vi "Logging.vi"(8 "error in (no error)":errorcluster, 11 "Node Ptr":T1 format="%.0x") -> (0 "error out":errorcluster)   [LabVIEW 2020, in "Ballard ARINC 429 System Explorer.lvlib" / "Implementation.lvlib"]
uses:
  Implementation.lvlib
  <vilib>/NI VeriStand/Custom Device API/Custom Device API.lvlib
  Scripting/Ballard/Ballard ARINC 429 Scripting.lvlib
  <vilib>/NI VeriStand/Custom Device API/Custom Device Item Ref.ctl
panel:
  in  "Log Messages?":bool
  in  "Log Directory":string
  in  "SHDocVw.IWebBrowser":refnum<k7>(container)
  in  "General Header":cluster{"Section Name":string}={"Section Name"="Ballard ARINC 429 - Logging"}
  in  "Description":string
  out "Name":string
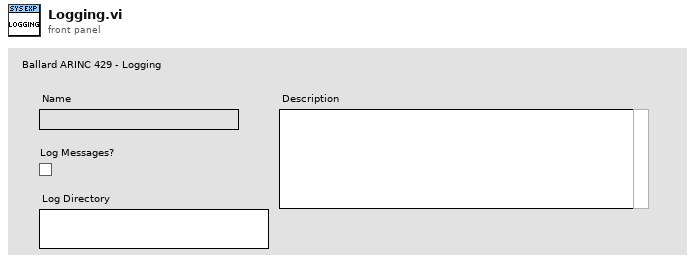
[diagram p1: front panel]
types:
  T1 = typedef "Custom Device API.lvlib/Custom Device Item Ref.ctl" = u64
  T2 = typedef "Custom Device API.lvlib/Custom Device Item Info.ctl" = cluster{"Name":string, "Is Channel":bool, "GUID":string, "Is Waveform":bool}
  T3 = typedef "Custom Device API.lvlib/Custom Device Commands.ctl" = enum16{"Default", "Item renamed", "Shutdown", "Dynamic button pressed"}
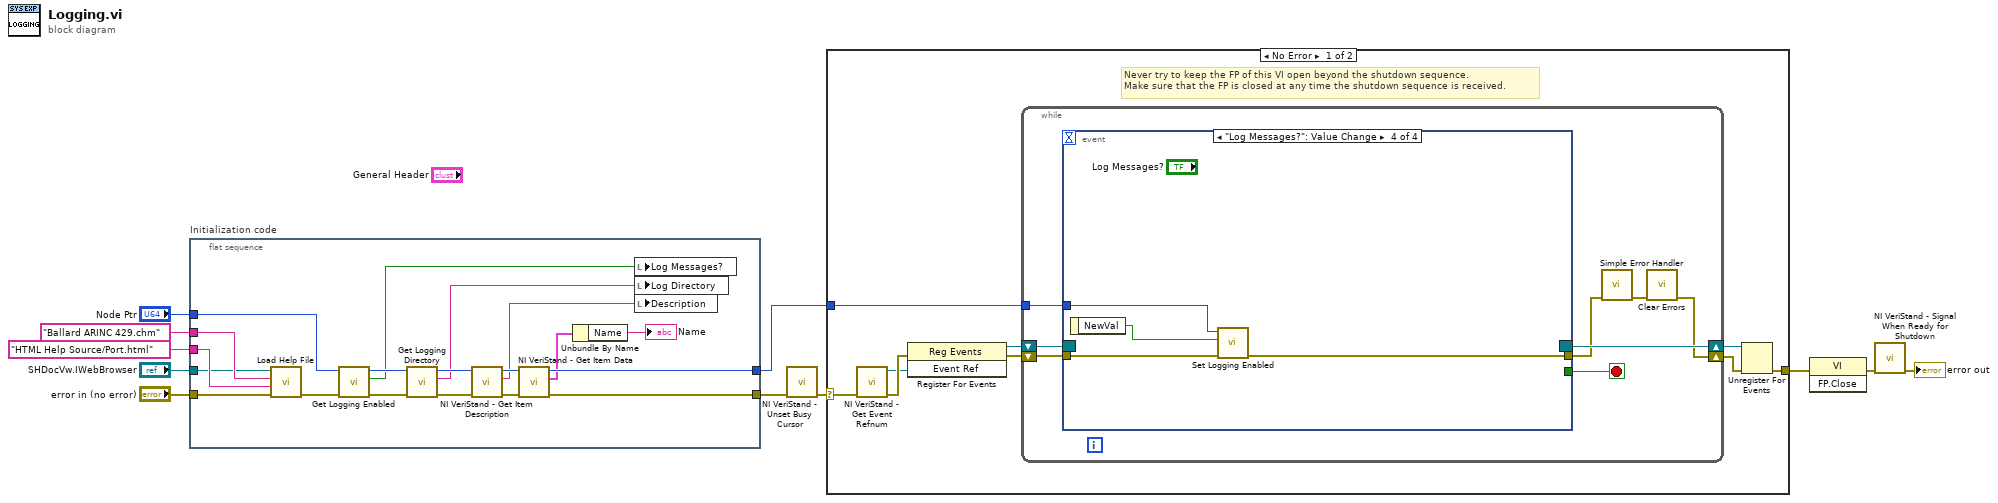
[diagram p0: block diagram]
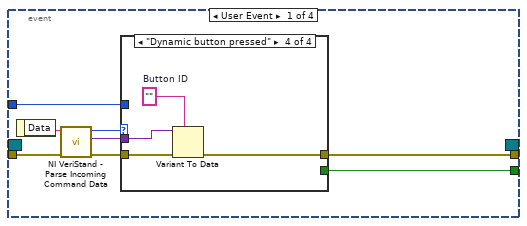
[diagram p2: hidden frame]
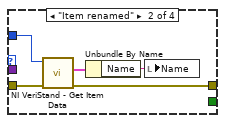
[diagram p4: hidden frame]
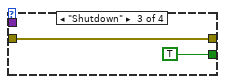
[diagram p5: hidden frame]
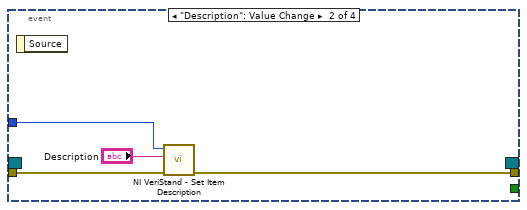
[diagram p6: hidden frame]
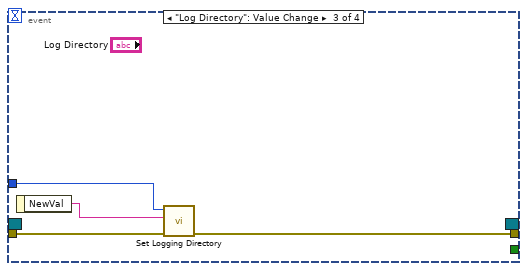
[diagram p7: hidden frame]
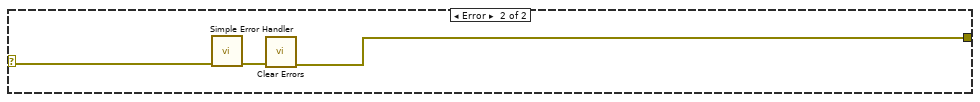
[diagram p8: hidden frame]
diagram:
  n1 = flat-sequence "Initialization code" {
    tunnel: "error in (no error)" -> [w24]
    tunnel: "Node Ptr" -> [w14]
    tunnel: [w26] -> w7
    tunnel: [w30] -> w4
    tunnel: "SHDocVw.IWebBrowser" -> [w21]
    tunnel: "HTML Help Source/Port.html" ("CD_CHM_Section") -> [w23]
    tunnel: "Ballard ARINC 429.chm" ("CD_CHM_FileName") -> [w22]
    frame #0 {
      n2 = call "Load Help File.vi"("error in (no error)"=w24, "HTML File to Load"=w23, "Main CHM File"=w22, "Browser"=w21) -> ("error out"=w18:errorcluster)  [unwired: 7 in]
      n3 = call "Get Logging Enabled.vi"("error in"=w18, "logging in"=w14) -> ("error out"=w15:errorcluster, "logging enabled"=w12:bool, "logging out"=w13:T1)  [unwired: 7 in]
      n4 = call "Get Logging Directory.vi"("error in"=w15, "logging in"=w13) -> ("error out"=w17:errorcluster, "directory"=w16:string, "logging out"=w19:T1)  [unwired: 7 in]
      n5 = call <vilib>:"NI VeriStand - Get Item Description.vi"("error in (no error)"=w17, "Item Ref in"=w19) -> ("error out"=w28:errorcluster, "Description"=w25:string, "Item Ref out"=w29:T1)  [unwired: 7 out]
      n6 = call <vilib>:"NI VeriStand - Get Item Data.vi"("error in (no error)"=w28, "Item Ref in"=w29) -> ("error out"=w26:errorcluster, "Item Info"=w27:T2, "Item Ref out"=w30:T1)  [unwired: 7 out]
      n7 = Unbundle By Name(w27) -> ("Name"=→"Name":string)
      n8 = local write "Log Messages?"(w12) -> ()
      n9 = local write "Log Directory"(w16) -> ()
      n10 = local write "Description"(w25) -> ()
    }
  }
  n11 = call <vilib>:"NI VeriStand - Unset Busy Cursor.vi"("error in (no error)"=w7) -> ("error out"=w6:errorcluster)  [unwired: 10 out]
  n12 = case shown="No Error" w6 {
    selector: w6 -> [w31 w82]
    tunnel: [w36 w80] -> w11
    tunnel: w4 -> [w32 _]
    frame No Error {
      # "Never try to keep the FP of this VI open beyond the shutdown sequence.\nMake sure that the FP is closed at any time the shutdown sequence is received."
      n13 = call <vilib>:"NI VeriStand - Get Event Refnum.vi"("error in (no error)"=w31) -> ("error out"=w39:errorcluster, "Event Ref"=w35:refnum<user-event>)  [unwired: 9 out]
      n14 = register-events(error in=w39, w35) -> (reference out=w33:refnum<event-registration>, error out=w34:errorcluster)  [unwired: 1 in]
      n15 = while {
        tunnel: w32 -> [w43]
        shift-right: [w40] -> w37
        shift-left: w34 -> [w46]
        shift-right: [w47] -> w38
        shift-left: w33 -> [w45]
        stop <- w44 stop-if-true
        n16 = event shown="[3] \"Log Messages?\": Value Change" {
          selector: w45 -> [_ _ _ _]
          dyn-events: [_ _ _ _] -> w47
          timeout: _ -> [_ _ _ _]
          tunnel: w46 -> [w55 w70 w75 w79]
          tunnel: [w51 _ _ _] -> w44
          tunnel: [w50 w69 w72 w78] -> w42
          tunnel: w43 -> [w49 w71 w74 w77]
          event User Event {
            n17 = event-data() -> ("Data"=w54:string)  [unwired: 1 out]
            n18 = call <vilib>:"NI VeriStand - Parse Incoming Command Data.vi"("error in (no error)"=w55, "Incoming data"=w54) -> ("error out"=w53:errorcluster, "Outgoing data"=w48:variant, "Action"=w52:T3)  [unwired: 7 out]
            n19 = case shown="\"Dynamic button pressed\"" w52 {
              tunnel: w53 -> [w56 w61 w62 w67]
              tunnel: [_ _ TRUE _] -> w51
              tunnel: [w56 w58 w62 w64] -> w50
              tunnel: w49 -> [_ w60 _ _]
              tunnel: w48 -> [_ _ _ w66]
              frame "Default", Default {
              }
              frame "Item renamed" {
                n20 = call <vilib>:"NI VeriStand - Get Item Data.vi"("error in (no error)"=w61, "Item Ref in"=w60) -> ("error out"=w58:errorcluster, "Item Info"=w59:T2)  [unwired: 8 out]
                n21 = Unbundle By Name(w59) -> ("Name"=w57:string)
                n22 = local write "Name"(w57) -> ()
              }
              frame "Shutdown" {
              }
              frame "Dynamic button pressed" {
                w65 = ""  # Button ID
                n23 = Variant To Data(error in=w67, type=w65, Variant=w66) -> (error out=w64:errorcluster)  [unwired: 1 out]
              }
            }
          }
          event "Description": Value Change {
            n24 = event-data() -> ()  [unwired: 2 out]
            n25 = call <vilib>:"NI VeriStand - Set Item Description.vi"("error in (no error)"=w70, "Description"="Description", "Item Ref in"=w71) -> ("error out"=w69:errorcluster)  [unwired: 8 out]
          }
          event "Log Directory": Value Change {
            n26 = event-data() -> ("NewVal"=w73:string)  [unwired: 1 out]
            n27 = call "Set Logging Directory.vi"("error in"=w75, "directory"=w73, "logging in"=w74) -> ("error out"=w72:errorcluster)  [unwired: 6 in, 1 out]
          }
          event "Log Messages?": Value Change {
            n28 = event-data() -> ("NewVal"=w76:bool)  [unwired: 1 out]
            n29 = call "Set Logging Enabled.vi"("error in"=w79, "logging enabled"=w76, "logging in"=w77) -> ("error out"=w78:errorcluster)  [unwired: 7 in, 1 out]
          }
        }
        n30 = call <vilib>:"Simple Error Handler.vi"("error in (no error)"=w42) -> ("error out"=w41:errorcluster)  [unwired: 1 in, 7 out]
        n31 = call <vilib>:"Clear Errors.vi"("error in (no error)"=w41) -> ("error out"=w40:errorcluster)  [unwired: 1 in, 5 out]
      }
      n32 = Unregister For Events(event registration refnum=w38, error in=w37) -> (error out=w36:errorcluster)
    }
    frame Error {
      n33 = call <vilib>:"Simple Error Handler.vi"("error in (no error)"=w82) -> ("error out"=w81:errorcluster)  [unwired: 1 in, 7 out]
      n34 = call <vilib>:"Clear Errors.vi"("error in (no error)"=w81) -> ("error out"=w80:errorcluster)  [unwired: 1 in, 5 out]
    }
  }
  n35 = invoke class="VI" method="FP.Close"(error in=w11) -> (error out=w10:errorcluster)  [unwired: 2 in, 2 out]
  n36 = call <vilib>:"NI VeriStand - Signal When Ready for Shutdown.vi"("error in (no error)"=w10) -> ("error out"=→"error out":errorcluster)  [unwired: 10 out]
